vi "WSVCAP SHL Host LL I2C Convert Bit Array to Channel Bytes.vi"(0 "Bit Array":u64[](array[numeric]) format="%06x") -> (4 "Read Data":u8[][](array[numeric]) format="%.0x")   [LabVIEW 2017]
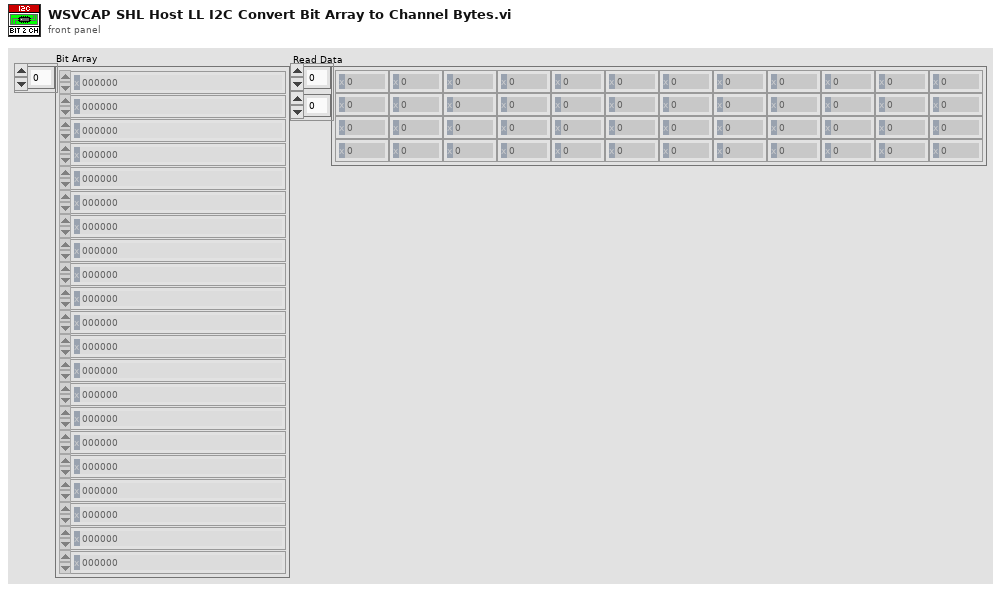
[diagram p1: front panel]
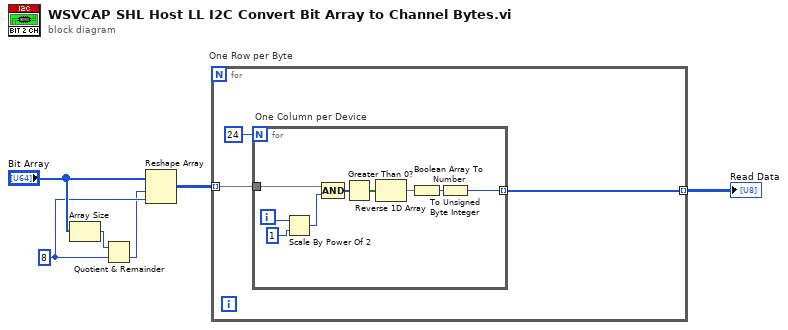
[diagram p0: block diagram]
diagram:
  w3 = 8 ("Read Data In")
  # "One Row per Byte"
  n1 = Array Size(array="Bit Array") -> (size(s)=w5:i32)
  n2 = Quotient & Remainder(x=w5, y=w3) -> (floor(x/y)=w2:i32)  [unwired: 1 out]
  n3 = Reshape Array("Bit Array", w2, w3) -> (w4:u64[][])
  n4 = for {
    tunnel: w4 -> [w9] mode=indexing
    tunnel: [w7] -> w1 mode=indexing
    # "One Column per Device"
    n5 = for {
      N: 24 -> [_]
      tunnel: w9 -> [w17]
      tunnel: [w13] -> w7 mode=indexing
      i -> [w12]
      n6 = Scale By Power Of 2(n=w12, x=u64 1) -> (x*2^n=w16:u64)
      n7 = Compound Arithmetic op=AND(w17, w16) -> (w15:u64[])
      n8 = Greater Than 0?(x=w15) -> (x > 0?=w11:bool[])
      n9 = Reverse 1D Array(array=w11) -> (reversed array=w10:bool[])
      n10 = Boolean Array To Number(Boolean array=w10) -> (number=w14:u32)
      n11 = To Unsigned Byte Integer(number=w14) -> (unsigned 8bit integer=w13:u8)
    }
  }
  "Read Data" <- w1
